vi "InitializeSDK.vi"   [LabVIEW 2010]
uses:
  Program Files/Meadowlark Optics/Blink 1920 HDMI/SDK/Blink_C_wrapper.dll
panel:
  # "Call this once at the beginning of your LabVIEW session\nto open communication to the SLM and load the calibration file. \nLabVIEW DOES NOT SUPPORT HIGH DPI AWARENESS, so your \nprimary monitor must be 100% to properly place images on the SLM"
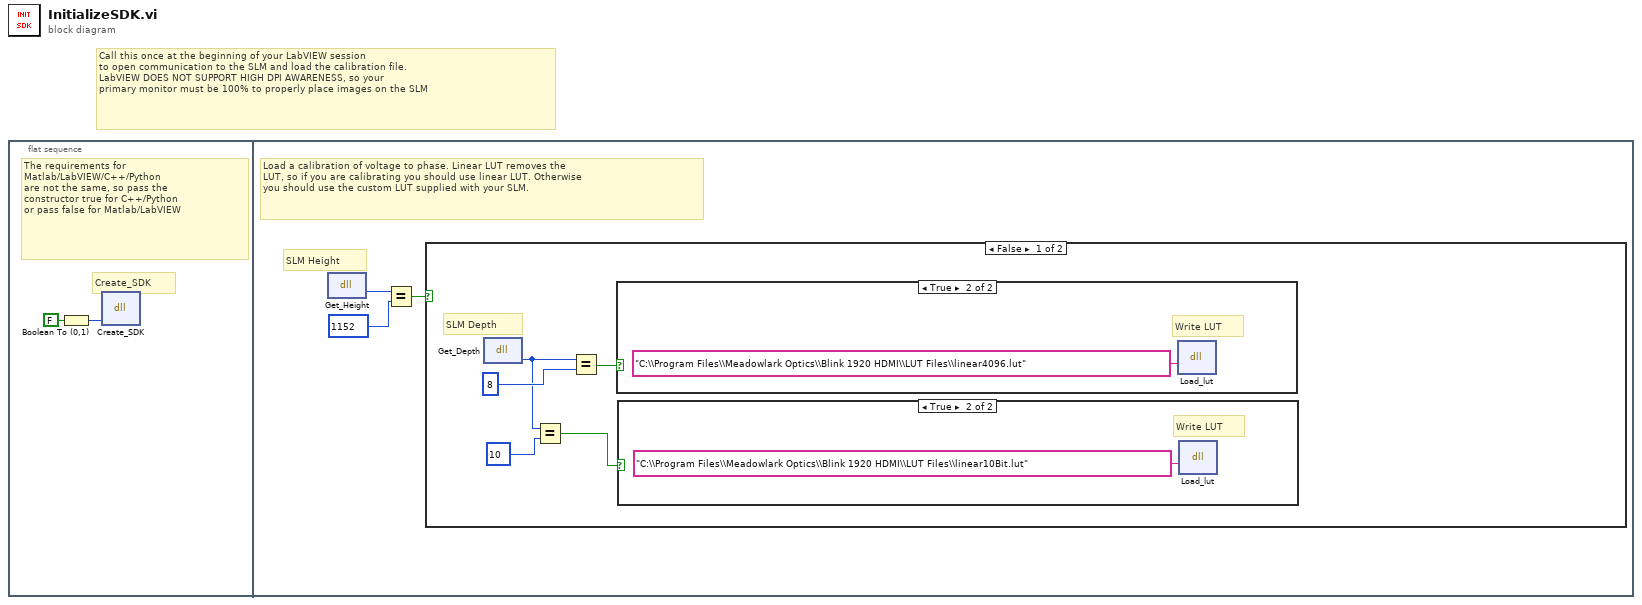
[diagram p0: block diagram]
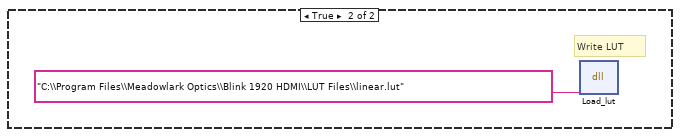
[diagram p4: hidden frame]
diagram:
  # "Call this once at the beginning of your LabVIEW session\nto open communication to the SLM and load the calibration file. \nLabVIEW DOES NOT SUPPORT HIGH DPI AWARENESS, so your \nprimary monitor must be 100% to properly place images on the SLM"
  n1 = flat-sequence {
    frame #0 {
      # "The requirements for \nMatlab/LabVIEW/C++/Python\nare not the same, so pass the \nconstructor true for C++/Python\nor pass false for Matlab/LabVIEW"
      # "Create_SDK"
      n2 = Boolean To (0,1)(Boolean=FALSE) -> (0, 1=w1:i16)
      n3 = dll-call lib="C:/Program Files/Meadowlark Optics/Blink 1920 HDMI/SDK/Blink_C_wrapper.dll" fn="Create_SDK"("arg1"=w1) -> ()  [unwired: 5 in, 2 out]
    }
    frame #1 {
      # "SLM Height"
      # "Load a calibration of voltage to phase. Linear LUT removes the \nLUT, so if you are calibrating you should use linear LUT. Otherwise \nyou should use the custom LUT supplied with your SLM."
      n4 = dll-call lib="C:/Program Files/Meadowlark Optics/Blink 1920 HDMI/SDK/Blink_C_wrapper.dll" fn="Get_Height"() -> ("return type"=w3:i32)  [unwired: 3 in, 2 out]
      n5 = Equal?(x=w3, y=1152) -> (x = y?=w5:bool)
      n6 = case shown="False" w5 {
        frame False {
          # "SLM Depth"
          n7 = dll-call lib="C:/Program Files/Meadowlark Optics/Blink 1920 HDMI/SDK/Blink_C_wrapper.dll" fn="Get_Depth"() -> ("return type"=w9:i32)  [unwired: 3 in, 2 out]
          n8 = Equal?(x=w9, y=10) -> (x = y?=w7:bool)
          n9 = Equal?(x=w9, y=8) -> (x = y?=w6:bool)
          n10 = case shown="True" w6 {
            frame False {
            }
            frame True {
              # "Write LUT"
              n11 = dll-call lib="C:/Program Files/Meadowlark Optics/Blink 1920 HDMI/SDK/Blink_C_wrapper.dll" fn="Load_lut"("Path"="C:\\Program Files\\Meadowlark Optics\\Blink 1920 HDMI\\LUT Files\\linear4096.lut") -> ()  [unwired: 5 in, 2 out]
            }
          }
          n12 = case shown="True" w7 {
            frame False {
            }
            frame True {
              # "Write LUT"
              n13 = dll-call lib="C:/Program Files/Meadowlark Optics/Blink 1920 HDMI/SDK/Blink_C_wrapper.dll" fn="Load_lut"("Path"="C:\\Program Files\\Meadowlark Optics\\Blink 1920 HDMI\\LUT Files\\linear10Bit.lut") -> ()  [unwired: 5 in, 2 out]
            }
          }
        }
        frame True {
          # "Write LUT"
          n14 = dll-call lib="C:/Program Files/Meadowlark Optics/Blink 1920 HDMI/SDK/Blink_C_wrapper.dll" fn="Load_lut"("Path"="C:\\Program Files\\Meadowlark Optics\\Blink 1920 HDMI\\LUT Files\\linear.lut") -> ()  [unwired: 5 in, 2 out]
        }
      }
    }
  }
